vi "CheckUpdate.vi"(10 "Установленная версия ПО":string, 11 "GitHub":bool) -> (3 "Последняя версия ПО":string)   [LabVIEW 2017]
uses:
  <vilib>/Platform/browser.llb/Open URL in Default Browser (string).vi
  Global_SNK3_HF.vi
panel:
  # "Проверка обновлений..."
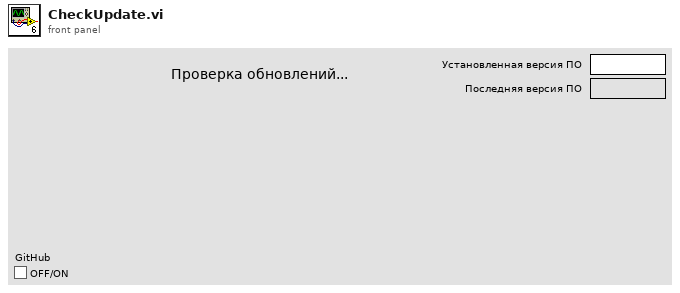
[diagram p1: front panel]
types:
  T1 = cluster{"published_at":timestamp, "Major":u32, "Minor":u32, "Fix":u32}
  T2 = cluster{"tag_name":string, "created_at":string, "updated_at":string, "published_at":string, "assets":cluster{"browser_download_url":string}[], "html_url":string}
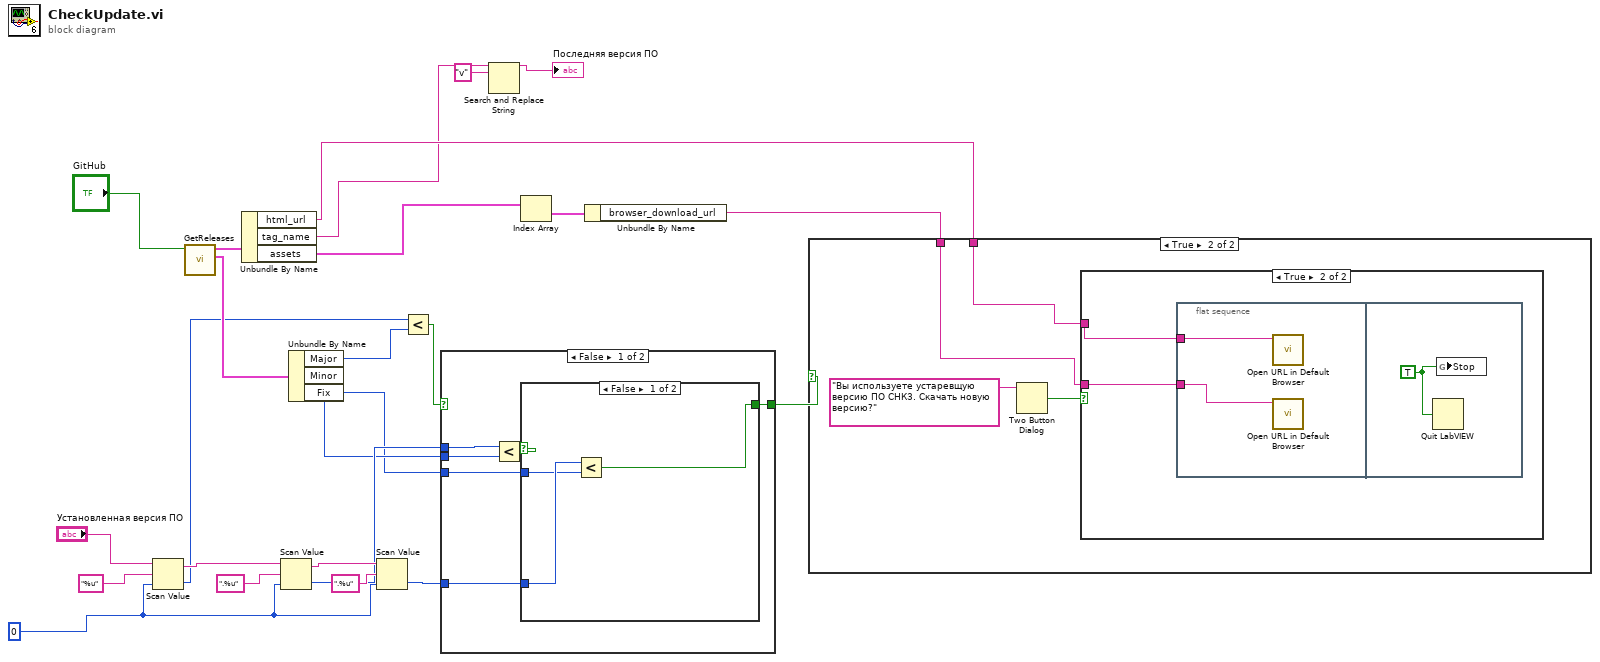
[diagram p0: block diagram]
diagram:
  w16 = u32 0 ("Fix")
  n1 = Scan Value(string="Установленная версия ПО", format string="%u", default (0 dbl)=w16) -> (output string=w21:string, value=w15:u32)
  n2 = call "GetReleases.vi"("GitHub"="GitHub") -> ("Info"=w23:T1, "infoReleases"=w25:T2)  [unwired: 9 in]
  n3 = Unbundle By Name(w25) -> ("html_url"=w4:string, "tag_name"=w3:string, "assets"=w7:cluster{"browser_download_url":string}[])
  n4 = Scan Value(string=w21, format string=".%u", default (0 dbl)=w16) -> (output string=w18:string, value=w12:u32)
  n5 = Unbundle By Name(w23) -> ("Major"=w14:u32, "Minor"=w11:u32, "Fix"=w10:u32)
  n6 = Scan Value(string=w18, format string=".%u", default (0 dbl)=w16) -> (value=w9:u32)  [unwired: 1 out]
  n7 = Less?(x=w15, y=w14) -> (x < y?=w13:bool)
  n8 = case shown="False" w13 {
    selector: w13 -> [_ w36]
    tunnel: w12 -> [w31 _]
    tunnel: w11 -> [w30 _]
    tunnel: w10 -> [w28 _]
    tunnel: w9 -> [w27 _]
    tunnel: [w26 w36] -> w8
    frame False {
      n9 = Less?(x=w31, y=w30) -> (x < y?=w29:bool)
      n10 = case shown="False" w29 {
        selector: w29 -> [_ w35]
        tunnel: w28 -> [w32 _]
        tunnel: w27 -> [w33 _]
        tunnel: [w34 w35] -> w26
        frame False {
          n11 = Less?(x=w33, y=w32) -> (x < y?=w34:bool)
        }
        frame True {
        }
      }
    }
    frame True {
    }
  }
  n12 = Search and Replace String(input string=w3, search string="v") -> (result string=→"Последняя версия ПО":string)  [unwired: 6 in, 3 out]
  n13 = Index Array(array=w7) -> (element=w6:cluster{"browser_download_url":string})  [unwired: 1 in]
  n14 = Unbundle By Name(w6) -> ("browser_download_url"=w5:string)
  n15 = case shown="True" w8 {
    tunnel: w5 -> [_ w39]
    tunnel: w4 -> [_ w37]
    frame False {
    }
    frame True {
      n16 = Two Button Dialog(message="Вы используете устаревщую  версию ПО СНК3. Скачать новую версию?") -> (T button?=w40:bool)  [unwired: 2 in]
      n17 = case shown="True" w40 {
        tunnel: w39 -> [_ w42]
        tunnel: w37 -> [_ w41]
        frame False {
        }
        frame True {
          n18 = flat-sequence {
            tunnel: w42 -> [w44]
            tunnel: w41 -> [w43]
            frame #0 {
              n19 = call-poly <vilib>:"Open URL in Default Browser.vi"("URL"=w43) -> ()  [unwired: 5 in, 2 out]
              n20 = call-poly <vilib>:"Open URL in Default Browser.vi"("URL"=w44) -> ()  [unwired: 5 in, 2 out]
            }
            frame #1 {
              w45 = TRUE ("Stop")
              n21 = Quit LabVIEW(quit? (T)=w45) -> ()
              n22 = global write "Global_SNK3_HF.vi" "Stop"(w45) -> ()
            }
          }
        }
      }
    }
  }
